vi "creat task.vi"(8 "error in":errorcluster) -> (0 "error out":errorcluster, 3 "task out":refnum<k21>)   [LabVIEW 2020]
uses:
  <vilib>/DAQmx/create/channels.llb/DAQmx Create Channel (CI-Frequency).vi
  <resource>/objmgr/daqmx.rc
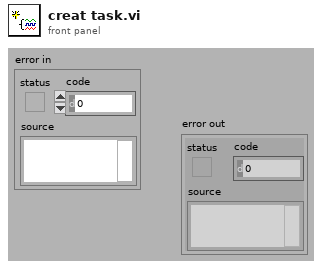
[diagram p1: front panel]
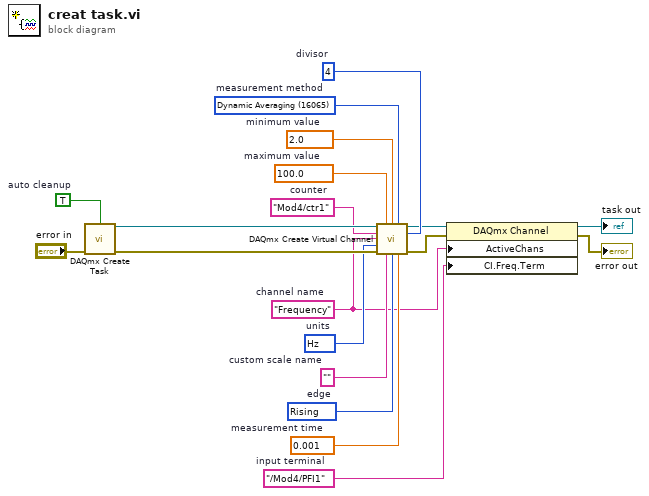
[diagram p0: block diagram]
diagram:
  w1 = 16065 items=["Low Frequency with 1 Counter"=10105, "High Frequency with 2 Counters"=10157, "Large Range with 2 Counters"=10205, "Dynamic Averaging"=16065]  # measurement method
  w2 = "/Mod4/PFI1"  # input terminal
  w7 = 10373 items=["Hz"=10373, "Ticks"=10304, "From Custom Scale"=10065]  # units
  w8 = 0.001  # measurement time
  w9 = u32 4  # divisor
  w10 = 10280 items=["Rising"=10280, "Falling"=10171]  # edge
  w3 = "Frequency"  # channel name
  w12 = ""  # custom scale name
  w13 = 2.0  # minimum value
  w14 = 100.0  # maximum value
  w15 = "Mod4/ctr1"  # counter
  w17 = TRUE  # auto cleanup
  n1 = call <vilib>:"DAQmx Create Task.vi"("auto cleanup"=w17, "error in"="error in") -> ("task out"=w16:refnum<k21>, "error out"=w18:errorcluster)  [unwired: 12 in]
  n2 = call-poly <vilib>:"DAQmx Create Virtual Channel.vi"("task in"=w16, "maximum value"=w14, "minimum value"=w13, "measurement method"=w1, "counter"=w15, "divisor"=w9, "name to assign"=w3, "units"=w7, "error in"=w18, "custom scale name"=w12, "starting edge"=w10, "measurement time"=w8) -> ("task out"=w5:refnum<k21>, "error out"=w11:errorcluster)  [unwired: 2 in]
  n3 = property class="DAQmx Channel"(reference=w5, error in=w11, "ActiveChans"=w3, "CI.Freq.Term"=w2) -> (reference out=→"task out":refnum<k21>, error out=→"error out":errorcluster)
